vi "merFISH_define_injections_procedure_list_names.vi"(4 "Buffer list":string[][](array[string]), 5 "error in":errorcluster, 6 "Injection procedure IN photobleaching":i32[][](array[numeric]), 7 "Injection procedure IN hybridization":i32[][](array[numeric])) -> (0 "Photobleaching name":string[](array[string]), 1 "Hybridization name":string[](array[string]), 2 "error out":errorcluster, 3 "Buffer selection list":string[][](array[string]))   [LabVIEW 2015]
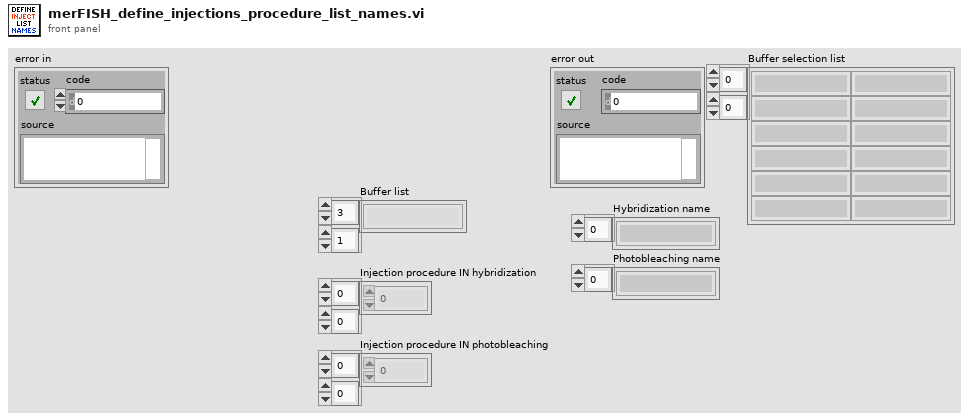
[diagram p1: front panel]
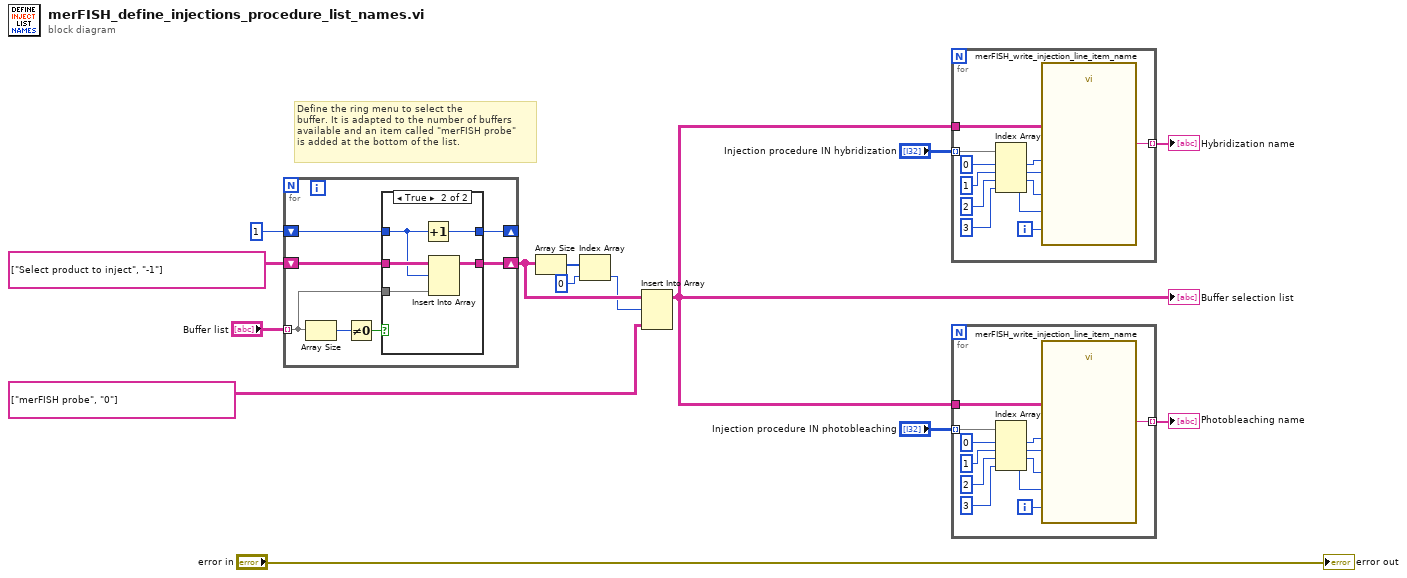
[diagram p0: block diagram]
diagram:
  # "Define the ring menu to select the \nbuffer. It is adapted to the number of buffers \navailable and an item called \"merFISH probe\"\nis added at the bottom of the list."
  n1 = for {
    tunnel: "Buffer list" -> [w17] mode=indexing
    shift-right: [w19] -> _
    shift-left: 1 ("dimension size") -> [w20]
    shift-right: [w18] -> w12
    shift-left: string[][] [["Select product to inject", "-1"]] ("initialized array") -> [w21]
    n2 = Array Size(array=w17) -> (size(s)=w16:i32)
    n3 = Not Equal To 0?(x=w16) -> (x != 0?=w15:bool)
    n4 = case shown="True" w15 {
      tunnel: w21 -> [w22 w28]
      tunnel: w17 -> [_ w27]
      tunnel: w20 -> [w23 w26]
      tunnel: [w23 w24] -> w19
      tunnel: [w22 w25] -> w18
      frame False {
      }
      frame True {
        n5 = Increment(x=w26) -> (x+1=w24:i32)
        n6 = Insert Into Array(array=w28, index (row)=w26, new element=w27) -> (w25:string[][])  [unwired: 1 in]
      }
    }
  }
  n7 = Array Size(array=w12) -> (size(s)=w4:i32[])
  n8 = Index Array(array=w4, index=0) -> (element=w3:i32)
  n9 = Insert Into Array(array=w12, index (row)=w3, new element=string[][] [["merFISH probe", "0"]] ("initialized array")) -> (w1:string[][])  [unwired: 1 in]
  "Buffer selection list" <- w1
  n10 = for {
    tunnel: "Injection procedure IN hybridization" -> [w39] mode=indexing
    tunnel: [w40] -> w10 mode=indexing
    tunnel: w1 -> [w35]
    i -> [w34]
    n11 = Index Array(array=w39, index #1=0 ("index"), index #2=1 ("index"), index #3=2 ("index"), index #4=3 ("index")) -> (element #1=w33:i32, element #2=w32:i32, element #3=w30:i32, element #4=w29:i32)
    n12 = call "merFISH_write_injection_line_item_name.vi"("Flow rate (µl/min)"=w30, "Select product"=w29, "Injection line number"=w34, "Buffer list"=w35, "Volume (µl)"=w32, "Pressure (mbar)"=w33) -> ("Task name"=w40:string)  [unwired: 3 in]
  }
  "Hybridization name" <- w10
  n13 = for {
    tunnel: "Injection procedure IN photobleaching" -> [w51] mode=indexing
    tunnel: [w52] -> w9 mode=indexing
    tunnel: w1 -> [w47]
    i -> [w46]
    n14 = Index Array(array=w51, index #1=0 ("index"), index #2=1 ("index"), index #3=2 ("index"), index #4=3 ("index")) -> (element #1=w45:i32, element #2=w44:i32, element #3=w42:i32, element #4=w41:i32)
    n15 = call "merFISH_write_injection_line_item_name.vi"("Flow rate (µl/min)"=w42, "Select product"=w41, "Injection line number"=w46, "Buffer list"=w47, "Volume (µl)"=w44, "Pressure (mbar)"=w45) -> ("Task name"=w52:string)  [unwired: 3 in]
  }
  "Photobleaching name" <- w9
  "error out" <- "error in"
